vi "Data Acqu (SubVI).vi"(4 "Period (s) in":dbl, 5 "R Offset in":dbl, 6 "Numeric":i32, 7 "IR Offset in":dbl, 8 "AI Ref In":T1, 9 "dt (ms) in":i64, 10 "Array in":dbl[](array[numeric]), 11 "Array 3":dbl[](array[numeric])) -> (0 "error out":errorcluster, 1 "Boolean":bool, 2 "Array out":dbl[](array[numeric]), 3 "Array 4":dbl[](array[numeric]))   [LabVIEW 2021]
uses:
  <vilib>/myRIO/Instrument Drivers/Onboard IO/AI/typedefs/AI Reference.ctl
  <vilib>/myRIO/Common/Instrument Driver Framework/Utilities/typedefs/myRIO Generic Hardware Reference.ctl
  <vilib>/myRIO/Common/Instrument Driver Framework/Utilities/typedefs/Hardware Version Enum.ctl
  <vilib>/myRIO/Common/Instrument Driver Framework/Utilities/typedefs/myRIO v1.0 Reference.ctl
  <vilib>/myRIO/Common/Instrument Driver Framework/Utilities/typedefs/Generic FPGA Reference.ctl
  <vilib>/myRIO/Common/Instrument Driver Framework/myRIO v1.0/AI/typedefs/AI Channels List.ctl
  <vilib>/myRIO/Common/Instrument Driver Framework/myRIO v1.0/AI/typedefs/AI Channels Enum.ctl
  <vilib>/myRIO/Common/Instrument Driver Framework/Utilities/typedefs/Analog Scaling Constants List.ctl
  <vilib>/myRIO/Common/Instrument Driver Framework/Utilities/typedefs/Analog Scaling Constants.ctl
  <vilib>/Utility/error.llb/Error Cluster From Error Code.vi
  <vilib>/myRIO/Common/Instrument Driver Framework/myRIO v1.0/AI/vis/myRIO v1.0 Read AI.vi
  <vilib>/myRIO/Instrument Drivers/Onboard IO/AI/AI.lvlib
panel:
  in  "error in (no error)":errorcluster
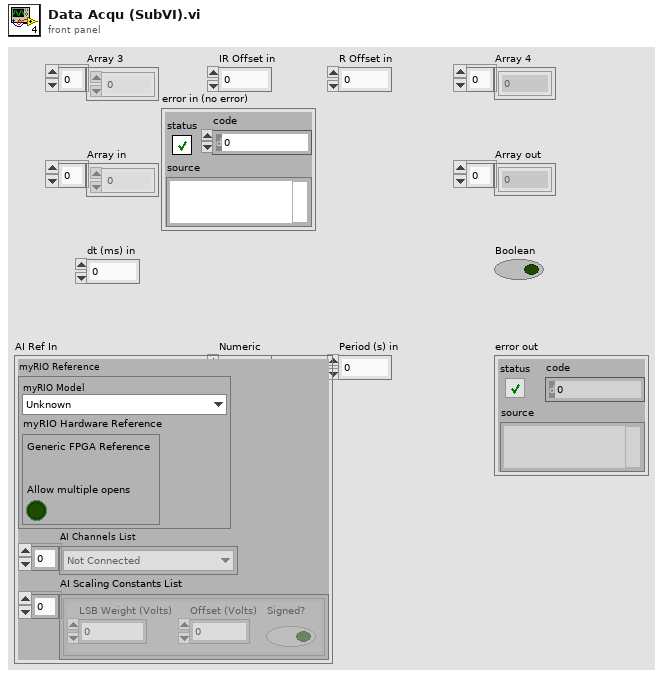
[diagram p1: front panel]
types:
  T1 = typedef "AI.lvlib/AI Reference.ctl" = cluster{"myRIO Reference":T2, "AI Channels List":T6, "AI Scaling Constants List":T8}
  T2 = typedef "myRIO Generic Hardware Reference.ctl" = cluster{"myRIO Model":T3, "myRIO Hardware Reference":T4}
  T3 = typedef "Hardware Version Enum.ctl" = enum16{"Unknown", "myRIO-1900", "myRIO-1950", "roboRIO", "NI ELVIS RIO CM", "ELVIS III"}
  T4 = typedef "myRIO v1.0 Reference.ctl" = cluster{"Generic FPGA Reference":T5, "Allow multiple opens":bool}
  T5 = typedef "Generic FPGA Reference.ctl" = refnum<k20>
  T6 = typedef "AI Channels List.ctl" = T7[]
  T7 = typedef "AI Channels Enum.ctl" = enum16{"Not Connected", "AudioIn/Left", "AudioIn/Right", "C/AI0", "C/AI1", "A/AI0", "A/AI1", "A/AI2", "A/AI3", "A/AI4", "A/AI5", "A/AI6", "A/AI7", "B/AI0", "B/AI1", "B/AI2", "B/AI3", "B/AI4", "B/AI5", "B/AI6", "B/AI7", "AI/AI0", "AI/AI1", "AI/AI2", "AI/AI3", "A/AI0 (DIFF)", "A/AI1 (DIFF)", "A/AI2 (DIFF)", "A/AI3 (DIFF)", "B/AI0 (DIFF)", "B/AI1 (DIFF)", "B/AI2 (DIFF)", "B/AI3 (DIFF)"}
  T8 = typedef "Analog Scaling Constants List.ctl" = T9[]
  T9 = typedef "Analog Scaling Constants.ctl" = cluster{"LSB Weight (Volts)":dbl, "Offset (Volts)":dbl, "Signed?":bool}
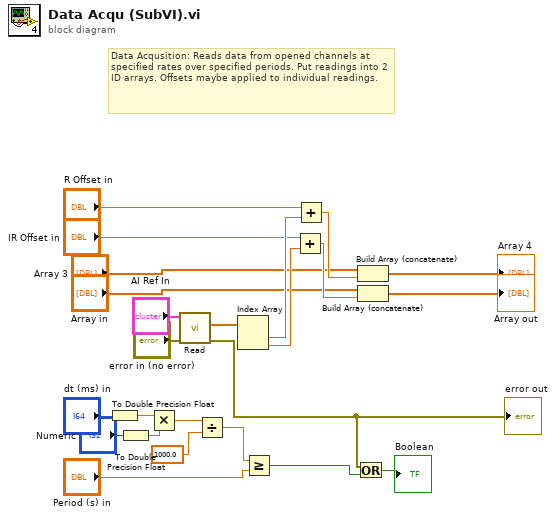
[diagram p0: block diagram]
diagram:
  # "Data Acqusition: Reads data from opened channels at specified rates over specified periods. Put readings into 2 ID arrays. Offsets maybe applied to individual readings."
  n1 = To Double Precision Float(number="dt (ms) in") -> (double precision float=w12:dbl)
  n2 = To Double Precision Float(number="Numeric") -> (double precision float=w10:dbl)
  n3 = Multiply(x=w12, y=w10) -> (x*y=w7:dbl)
  n4 = call <vilib>:"Read.vi"("error in (no error)"="error in (no error)", "AI Ref In"="AI Ref In") -> ("error out"=w23:errorcluster, "Values"=w15:dbl[])  [unwired: 7 in, 1 out]
  "error out" <- w23
  n5 = Divide(x=w7, y=1000.0) -> (x/y=w13:dbl)
  n6 = Index Array(array=w15) -> (element #1=w18:dbl, element #2=w19:dbl)  [unwired: 2 in]
  n7 = Greater Or Equal?(x=w13, y="Period (s) in") -> (x >= y?=w22:bool)
  n8 = Add(x="IR Offset in", y=w19) -> (x+y=w21:dbl)
  n9 = Add(x="R Offset in", y=w18) -> (x+y=w20:dbl)
  n10 = Or(x=w23, y=w22) -> (x .or. y?=→"Boolean":bool)
  n11 = Build Array (concatenate)("Array 3", w20) -> (→"Array 4":dbl[])
  n12 = Build Array (concatenate)("Array in", w21) -> (→"Array out":dbl[])
